vi "Write Coded binary.vi"(8 "error in":errorcluster, 10 "filter":u8, 11 "cPAS Data in":refnum<class "cPAS Data.lvclass">) -> (0 "error out":errorcluster, 3 "cPAS Data out":refnum<class "cPAS Data.lvclass">)   [LabVIEW 2012, in "cPAS Data.lvclass"]
uses:
  cPAS Data.lvclass
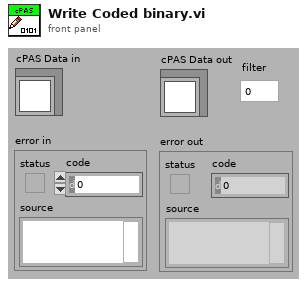
[diagram p1: front panel]
types:
  T1 = enum16{"big-endian, network order", "native, host order", "little-endian"}
  T2 = cluster{"24V":sgl, "+15V":sgl, "- 15V":sgl, "12V":sgl, "Aux Volt":sgl}
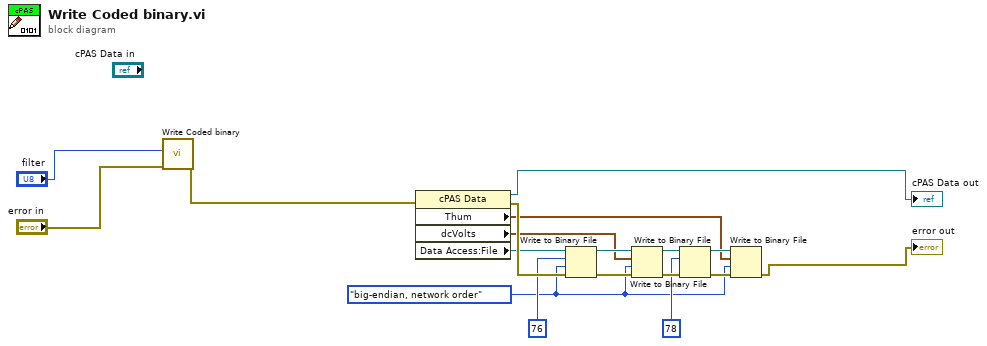
[diagram p0: block diagram]
diagram:
  w4 = T1."big-endian, network order" ("byte order (0:big-endian, network order)")
  n1 = call-parent "Write Coded binary.vi"("error in"="error in", "filter"="filter") -> ("error out"=w3:errorcluster)  [unwired: 8 in, 1 out]
  n2 = property class="cPAS Data"(error in=w3) -> (reference out=→"cPAS Data out":refnum<class "cPAS Data.lvclass">, error out=w16:errorcluster, "Thum"=w5:cluster{"Hum 1":sgl, "Hum 2":sgl}, "dcVolts"=w6:T2, "Data Access:File"=w7:refnum<file>)  [unwired: 1 in]
  n3 = Write to Binary File(file (use dialog)=w7, data=u8 76, error in=w16, 9:w4) -> (refnum out=w14:refnum<file>, error out=w13:errorcluster)  [unwired: 2 in, 1 out]
  n4 = Write to Binary File(file (use dialog)=w14, data=w6, error in=w13, 9:w4) -> (refnum out=w12:refnum<file>, error out=w11:errorcluster)  [unwired: 2 in, 1 out]
  n5 = Write to Binary File(file (use dialog)=w12, data=u8 78, error in=w11) -> (refnum out=w9:refnum<file>, error out=w8:errorcluster)  [unwired: 3 in, 1 out]
  n6 = Write to Binary File(file (use dialog)=w9, data=w5, error in=w8, 9:w4) -> (error out=→"error out":errorcluster)  [unwired: 2 in, 2 out]
